vi "Ethernet IP Global Strings.vi"() -> ()   [LabVIEW 2023, in "Ethernet IP Custom Device Custom Device.lvlib"]
uses:
  Ethernet IP Custom Device Custom Device.lvlib
panel:
  in  "Patth to Assembly Import file":string="Patth to Assembly Import file"
  in  "Attribute Info":string="Attribute Info"
  in  "Message Type":string="Message Type"
  in  "Path to L5K file":string="Path to L5K file"
  in  "Update Rate":string="Update Rate"
  in  "Tag Name":string="Tag Name"
  in  "Input?":string="Data Type"
  in  "Data Type":string="Data Type"
  in  "Network Path":string="Network Path"
  in  "Timeout":string="Timeout"
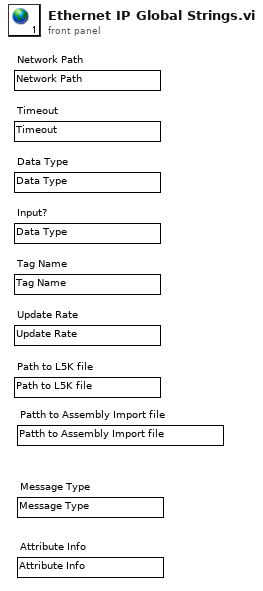
[diagram p1: front panel]
diagram:
